vi "H5LTmake_dataset_float.vi"(2 "SGL Array":variant, 3 "loc_id":i32, 7 "name":string, 9 "error in (no error)":errorcluster) -> (6 "error out":errorcluster)   [LabVIEW 2009]
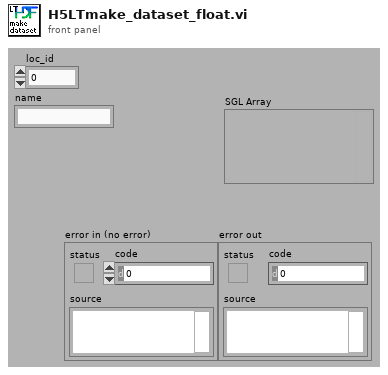
[diagram p1: front panel]
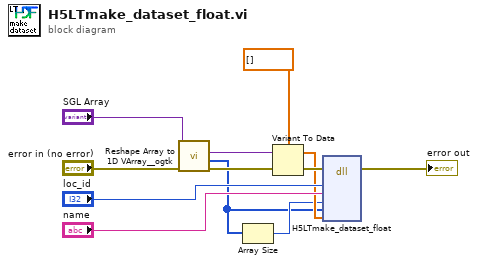
[diagram p0: block diagram]
diagram:
  n1 = call <userlib>:"Reshape Array to 1D VArray__ogtk.vi"("error in (no error)"="error in (no error)", "MultiD Array"="SGL Array") -> ("error out"=w5:errorcluster, "Size(s)"=w1:u32[], "1D VArray"=w3:variant)  [unwired: 7 in]
  n2 = Array Size(array=w1) -> (size(s)=w2:i32)
  n3 = Variant To Data(error in=w5, Variant=w3, type=sgl[] [] ("buffer")) -> (error out=w9:errorcluster, data=w7:sgl[])
  n4 = dll-call lib="hdf5_hldll" fn="H5LTmake_dataset_float"(error in=w9, "loc_id"="loc_id", "name"="name", "rank"=w2, "dims"=w1, "buffer"=w7) -> (error out=→"error out":errorcluster)  [unwired: 8 in, 1 out]
